vi "S-BoxLookupArray1D.vi"(11 "In":u8[](array[numeric])) -> (3 "Out":u8[](array[numeric]))   [LabVIEW 2020, in "Encryption.lvlib"]
doc: "Performs the S-box lookup for an 1D array.\n\n(c) Ton Plomp, 2011\nTHIS SOFTWARE IS PROVIDED AS IS, AND ANY WARRANTY IS REJECTED"
uses:
  Encryption.lvlib
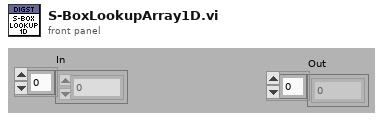
[diagram p1: front panel]
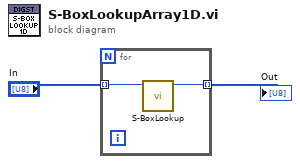
[diagram p0: block diagram]
diagram:
  n1 = for {
    tunnel: "In" -> [w4] mode=indexing
    tunnel: [w3] -> w1 mode=indexing
    n2 = call "S-BoxLookup.vi"("Value-In"=w4) -> ("LookUp-Out"=w3:u8)  [unwired: 10 in]
  }
  "Out" <- w1
